vi "GVSMain Sub Window Global.vi"() -> ()   [LabVIEW 2013]
uses:
  <vilib>/Utility/miscctls.llb/LVRectTypeDef.ctl
panel:
  in  "TitlebarHalfInactiveColor Graph":u32(colorbox)=16860
  in  "TitlebarTextColorInActive Graph":u32(colorbox)=16860
  in  "TitlebarInactiveColor Graph":u32(colorbox)=16860
  in  "TitlebarTextColorActive Graph":u32(colorbox)=16860
  in  "TitlebarActiveColor Graph":u32(colorbox)=16860
  in  "StepSetup Panel":u32(colorbox)=16860
  in  "cMsgProjectList":T1
  out "bProjectRun":bool
  in  "DBGLevel":string="LOG_OUT_LEVEL_1"
  in  "sProjectLoad":string
  in  "Pause Enable":u32(colorbox)=16860
  in  "Pause Disable":u32(colorbox)=16860
  out "VIBridge":refnum<vi>
  in  "TitlebarHalfInactiveColor":u32(colorbox)=16860
  in  "nDefaultSpliterPos":i32
  in  "sTaskWSYSTEM":string
  in  "cActionWSYSTEM":T2
  in  "sActiveWinTitle":string
  in  "g_TXTextControl":refnum<k7>
  out "gbDocumentStop":bool
  out "gbDocumentChange":bool
  out "gbMsg":bool
  out "bKTHDrawOK":bool
  in  "VIListDataView":string
  out "bStatusTemp":bool
  in  "gWorkPath":path
  in  "VIstuDoc":T3
  in  "VIListDoc":T4(array[cluster])
  in  "gOpenedVIs":string[](array[string])
  in  "gStop":bool
  in  "sWsysVersion":string
  in  "tWinType":T5 {"FOCUS_HIDE" format="%.0x"; "FOCUS_SHOW" format="%.0x"; "DOCK_DISABLE" format="%.0x"; "DOCK_ENABLE" format="%.0x"; "CLOSE_CLOSE" format="%.0x"; "CLOSE_HIDE" format="%.0x"}
  in  "cSave":T7
  in  "MinimizeState":T8(ring)=enum."Minimized"
  in  "MainTabID":i32
  out "MainTabVI":refnum<vi>
  out "MsgProVI":refnum<vi>
  out "gMouseButton":bool
  in  "Virtual_sPos":string
  out "DebugState":bool
  in  "tPage":T9
  in  "gMousePos":T10
  in  "CounterSpliter":i32
  in  "CounterActive":i32
  in  "cSpliter":T11
  in  "tSpliter":T12
  in  "MainFrame_nID":i32
  out "DockingState":bool
  in  "tFrame":T13
  in  "cFrame":T14
  out "MainFrame_VIRef":refnum<vi>
  out "ActiveVI":refnum<vi>
  in  "VritualDockWID":i32
  out "VritualDockVI":refnum<vi>
  out "MarkVisible":bool
  out "MarkVIs":refnum<vi>[](array[refnum])
  out "VritualVI":refnum<vi>
  out "VirtualVisible":bool
  out "Operator State":bool[](array[boolean])
  in  "Main View SubPanel":refnum<vi>
  in  "Main Pane Ref":refnum<vi>
  in  "Main Menu Refnum":refnum<k9>
  out "RunState":bool
  out "Main VI Ref":refnum<vi>
  in  "TitlebarTextColorInActive":u32(colorbox)=16860
  in  "TitlebarInactiveColor":u32(colorbox)=16860
  in  "ActiveWID":i32
  in  "TitlebarTextColorActive":u32(colorbox)=16860
  in  "TitlebarActiveColor":u32(colorbox)=16860
  in  "CounterWID":i32
  in  "Graph Cluster":T15
  # "GVSMain Splitter Global"
  # "\"\":No out Log\nLOG_OUT_LEVEL_1:level 1 log out"
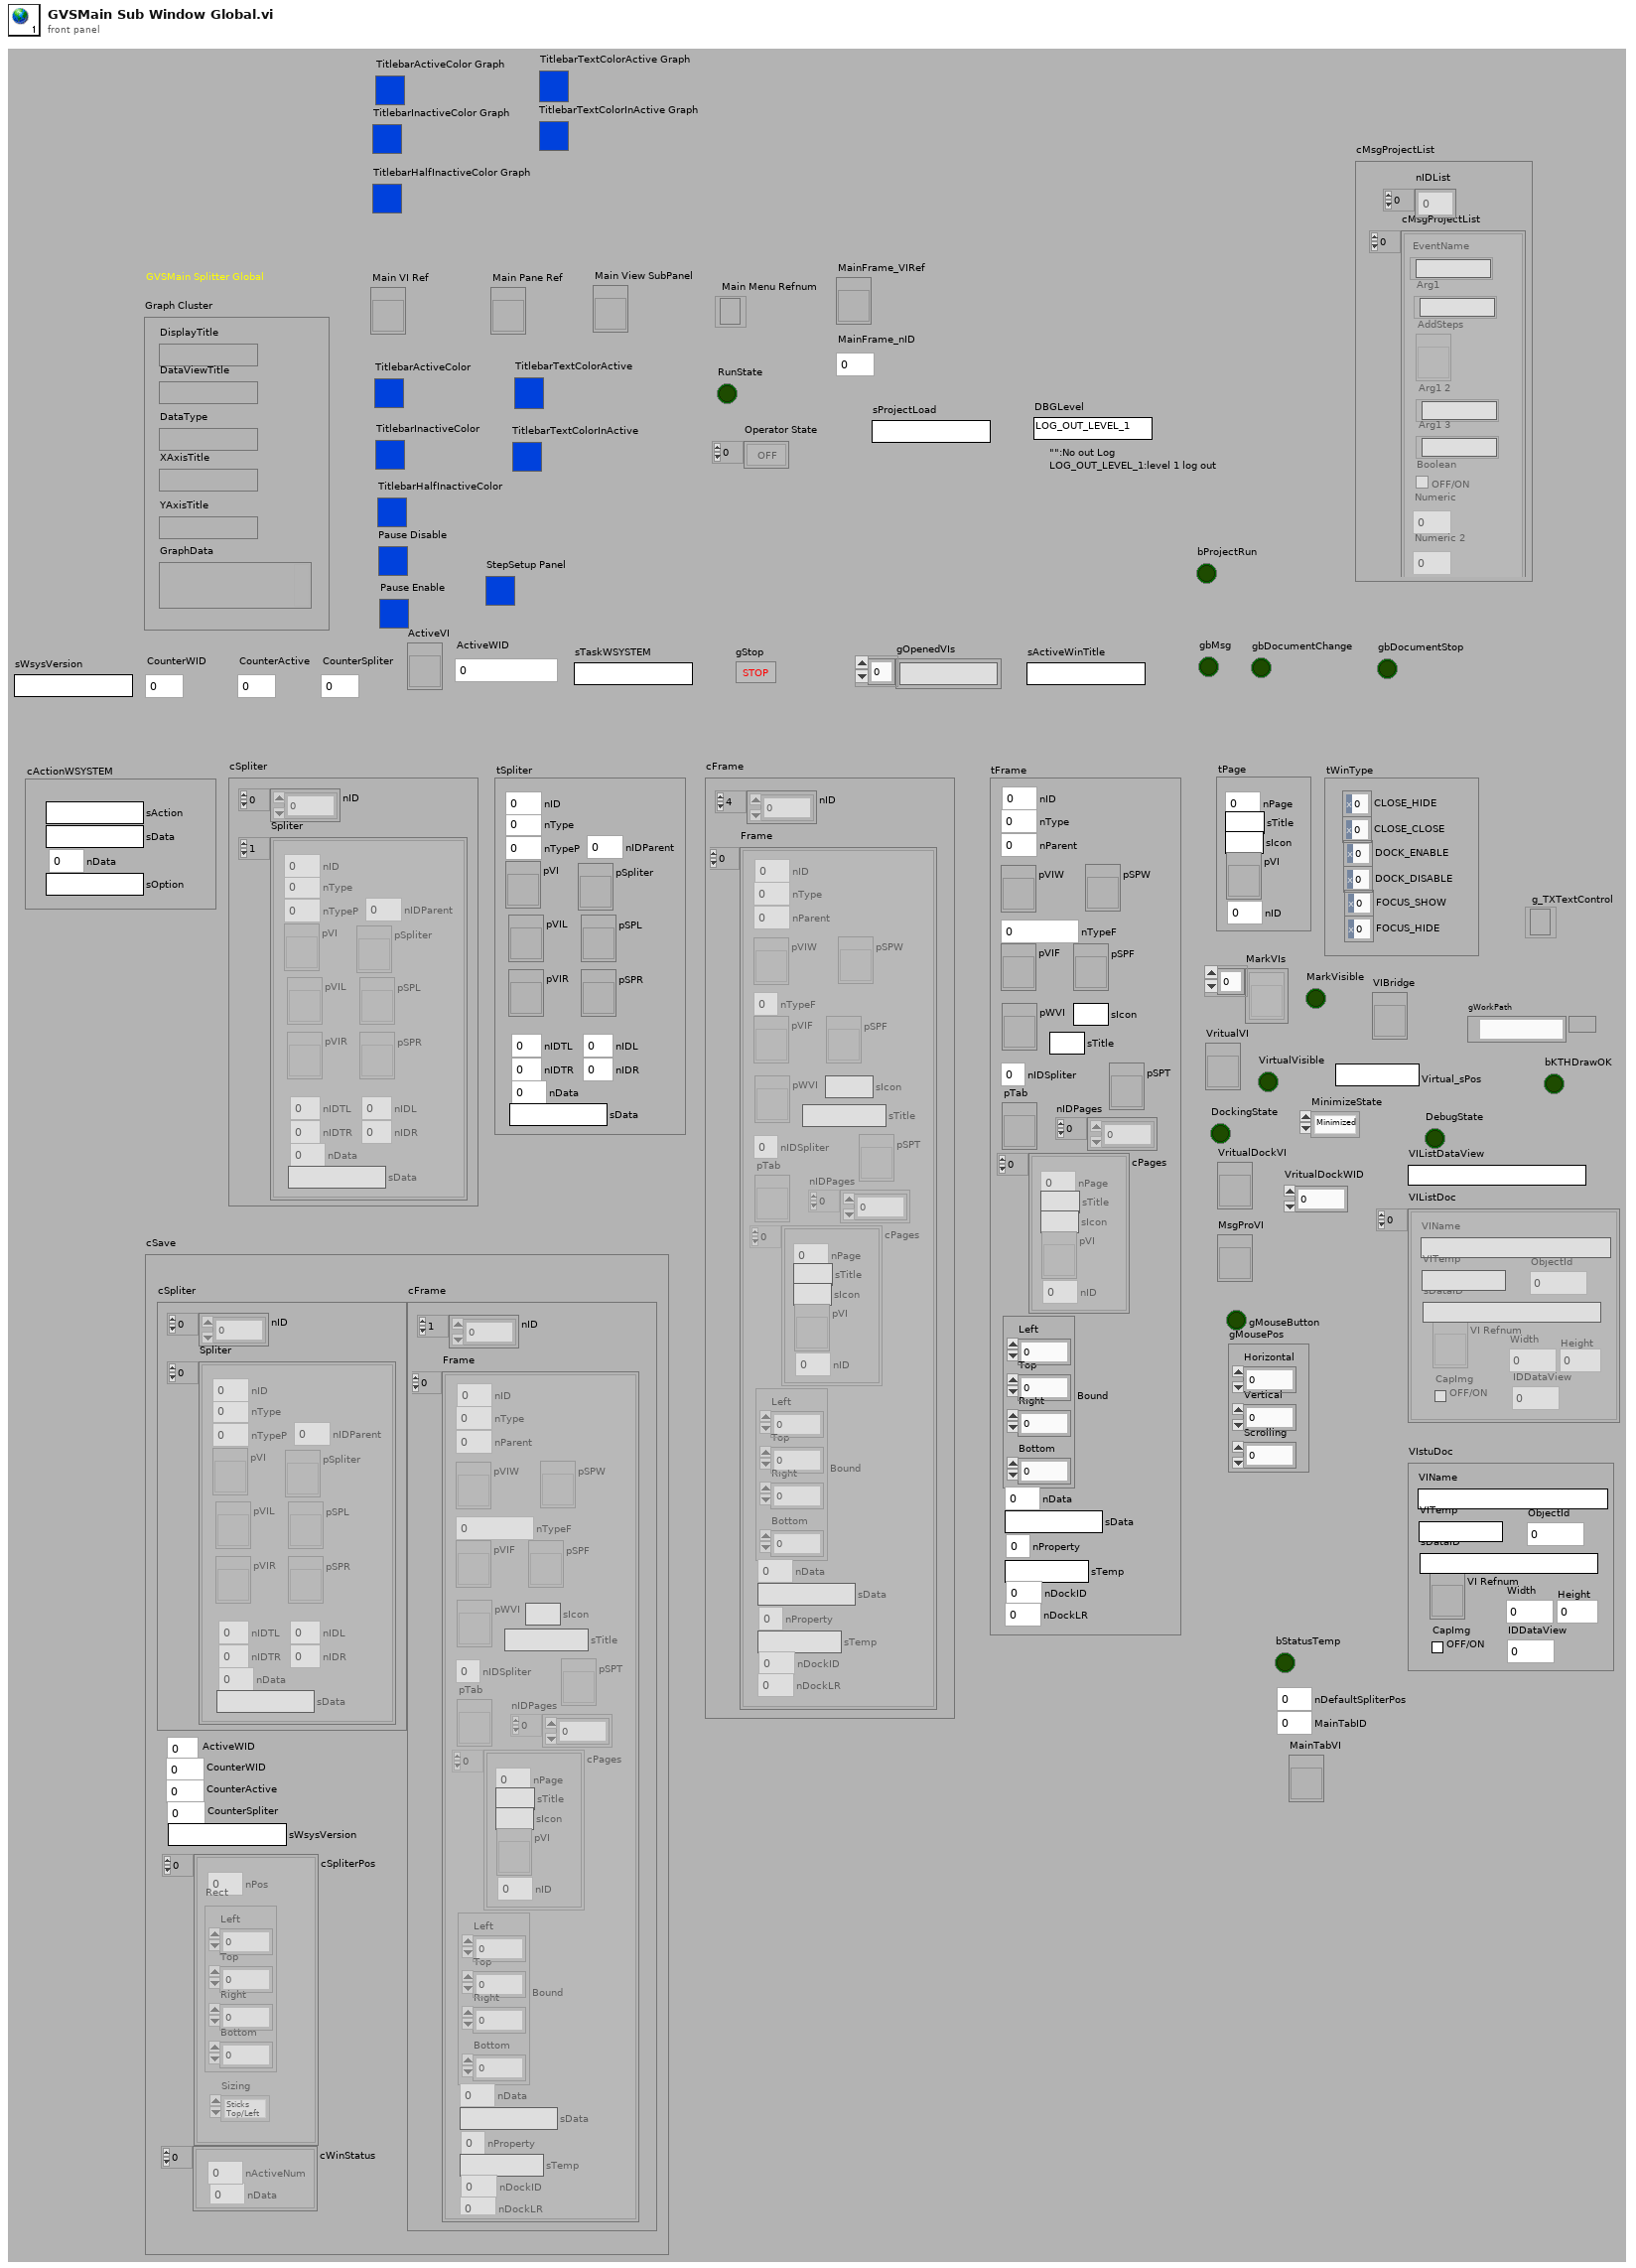
[diagram p1: front panel]
types:
  T1 = cluster{"cMsgProjectList":cluster{"EventName":string, "Arg1":string, "Numeric":u16, "Numeric 2":u16, "AddSteps ":refnum<vi>, "Arg1 2":string, "Arg1 3":string, "Boolean":bool}[], "nIDList":i32[]}
  T2 = cluster{"nData":i32, "sData":string, "sAction":string, "sOption":string}
  T3 = cluster{"VIName":string, "VI Refnum":refnum<vi>, "sDataID":string, "ObjectId":i16, "VITemp":string, "Width":i16, "Height":i16, "CapImg":bool, "IDDataView":i16}
  T4 = cluster{"VIName":string, "VI Refnum":refnum<vi>, "sDataID":string, "ObjectId":i16, "VITemp":string, "Width":i16, "Height":i16, "CapImg":bool, "IDDataView":i16}[]
  T5 = cluster{"CLOSE_HIDE":i32, "CLOSE_CLOSE":i32, "DOCK_ENABLE":i32, "DOCK_DISABLE":i32, "FOCUS_SHOW":i32, "FOCUS_HIDE":i32}
  T6 = typedef "LVRectTypeDef.ctl" = cluster{"Left":i16, "Top":i16, "Right":i16, "Bottom":i16}
  T7 = cluster{"cFrame":cluster{"nID":i32[], "Frame":cluster{"nType":i32, "nParent":i32, "pVIW":refnum<vi>, "pSPW":refnum<vi>, "nTypeF":i32, "pVIF":refnum<vi>, "pSPF":refnum<vi>, "nIDSpliter":i32, "nProperty":i32, "Bound":T6, "nID":i32, "nData":i32, "sData":string, "pWVI":refnum<vi>, "sTitle":string, "cPages":cluster{"nPage":i32, "sTitle":string, "sIcon":string, "pVI":refnum<vi>, "nID":i32}[], "pTab":refnum<vi>, "nIDPages":i32[], "pSPT":refnum<vi>, "sTemp":string, "nDockID":i32, "nDockLR":i32, "sIcon":string}[]}, "cSpliter":cluster{"nID":i32[], "Spliter":cluster{"nType":i32, "nTypeP":i32, "pVI":refnum<vi>, "pSpliter":refnum<vi>, "pSPL":refnum<vi>, "pVIL":refnum<vi>, "pSPR":refnum<vi>, "pVIR":refnum<vi>, "nIDTL":i32, "nIDL":i32, "nIDTR":i32, "nIDR":i32, "nID":i32, "nIDParent":i32, "nData":i32, "sData":string}[]}, "ActiveWID":i32, "cSpliterPos":cluster{"nPos":i32, "Rect":T6, "Sizing":enum16{"Sticks Top/Left", "Sticks Bottom/Right", "Proportional"}}[], "CounterWID":i32, "CounterActive":i32, "CounterSpliter":i32, "cWinStatus":cluster{"nData":i32, "nActiveNum":i32}[], "sWsysVersion":string}
  T8 = enum32{"Invalid", "Standard", "Closed", "Hidden", "Minimized", "Maximized"}
  T9 = cluster{"nPage":i32, "sTitle":string, "sIcon":string, "pVI":refnum<vi>, "nID":i32}
  T10 = cluster{"Horizontal":i32, "Vertical":i32, "Scrolling":i32}
  T11 = cluster{"nID":i32[], "Spliter":cluster{"nType":i32, "nTypeP":i32, "pVI":refnum<vi>, "pSpliter":refnum<vi>, "pSPL":refnum<vi>, "pVIL":refnum<vi>, "pSPR":refnum<vi>, "pVIR":refnum<vi>, "nIDTL":i32, "nIDL":i32, "nIDTR":i32, "nIDR":i32, "nID":i32, "nIDParent":i32, "nData":i32, "sData":string}[]}
  T12 = cluster{"nType":i32, "nTypeP":i32, "pVI":refnum<vi>, "pSpliter":refnum<vi>, "pSPL":refnum<vi>, "pVIL":refnum<vi>, "pSPR":refnum<vi>, "pVIR":refnum<vi>, "nIDTL":i32, "nIDL":i32, "nIDTR":i32, "nIDR":i32, "nID":i32, "nIDParent":i32, "nData":i32, "sData":string}
  T13 = cluster{"nType":i32, "nParent":i32, "pVIW":refnum<vi>, "pSPW":refnum<vi>, "nTypeF":i32, "pVIF":refnum<vi>, "pSPF":refnum<vi>, "nIDSpliter":i32, "nProperty":i32, "Bound":T6, "nID":i32, "nData":i32, "sData":string, "pWVI":refnum<vi>, "sTitle":string, "cPages":cluster{"nPage":i32, "sTitle":string, "sIcon":string, "pVI":refnum<vi>, "nID":i32}[], "pTab":refnum<vi>, "nIDPages":i32[], "pSPT":refnum<vi>, "sTemp":string, "nDockID":i32, "nDockLR":i32, "sIcon":string}
  T14 = cluster{"nID":i32[], "Frame":cluster{"nType":i32, "nParent":i32, "pVIW":refnum<vi>, "pSPW":refnum<vi>, "nTypeF":i32, "pVIF":refnum<vi>, "pSPF":refnum<vi>, "nIDSpliter":i32, "nProperty":i32, "Bound":T6, "nID":i32, "nData":i32, "sData":string, "pWVI":refnum<vi>, "sTitle":string, "cPages":cluster{"nPage":i32, "sTitle":string, "sIcon":string, "pVI":refnum<vi>, "nID":i32}[], "pTab":refnum<vi>, "nIDPages":i32[], "pSPT":refnum<vi>, "sTemp":string, "nDockID":i32, "nDockLR":i32, "sIcon":string}[]}
  T15 = cluster{"DisplayTitle":string, "DataViewTitle":string, "DataType":string, "XAxisTitle":string, "YAxisTitle":string, "GraphData":variant}
diagram:
